vi "uc480_SimpleLive_MultiCamera.vi"() -> ()   [LabVIEW 2011]
uses:
  C:/Program Files/Thorlabs/Scientific Imaging/DCx Camera Support/Develop/DotNet/uc480DotNet.dll
  Develop/DotNet/uc480DotNet.dll
panel:
  in  "Init Camera 2":bool
  in  "Exit Camera 2":bool
  out "Error Out 2":errorcluster caption="error"
  out "Bits/Pixel 2":i32=8
  out "Width":i32=8
  out "Height Height 2":i32=8
  out "Serial Number 2":string
  in  "Camera ID 2":i32
  out "Image second camera":picture
  out "Image first camera":picture
  in  "Camera ID 1":i32
  out "Serial Number 1":string
  out "Height Height":i32=8
  out "Width":i32=8
  out "Bits/Pixel":i32=8
  out "Error Out 1":errorcluster caption="error"
  in  "Exit Camera":bool
  in  "Init Camera":bool
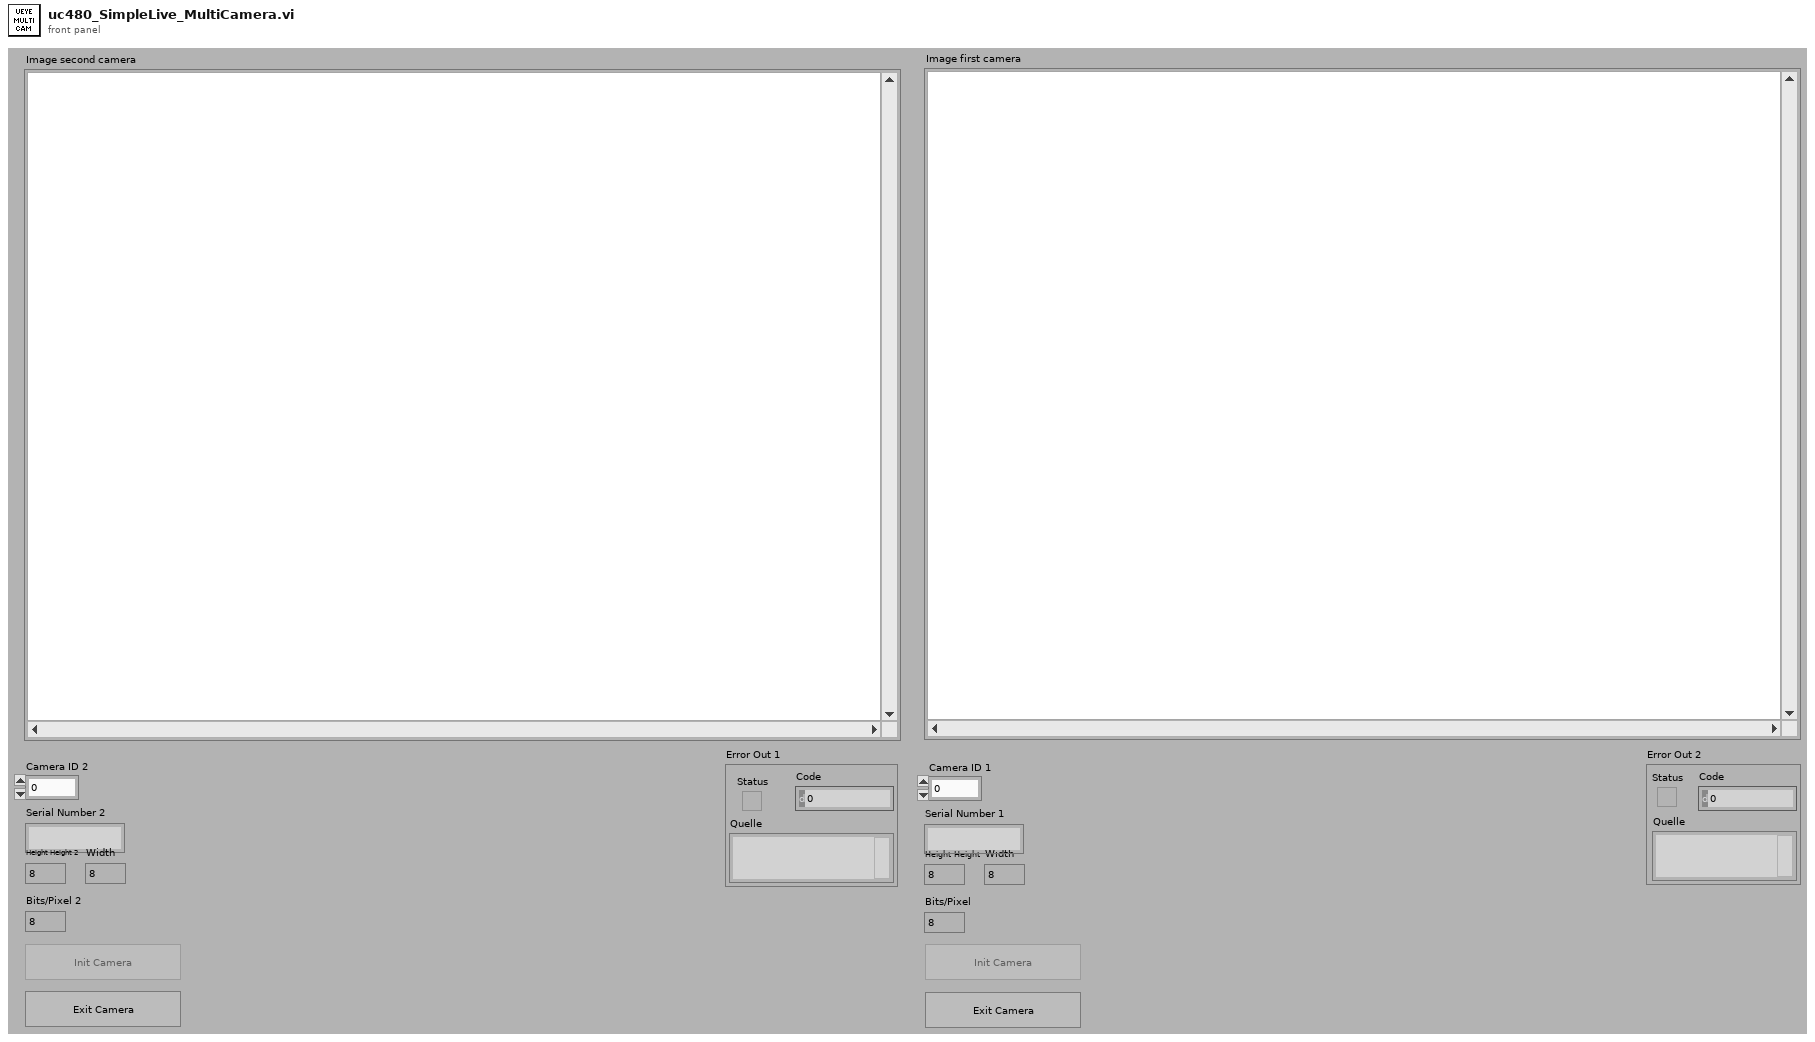
[diagram p1: front panel]
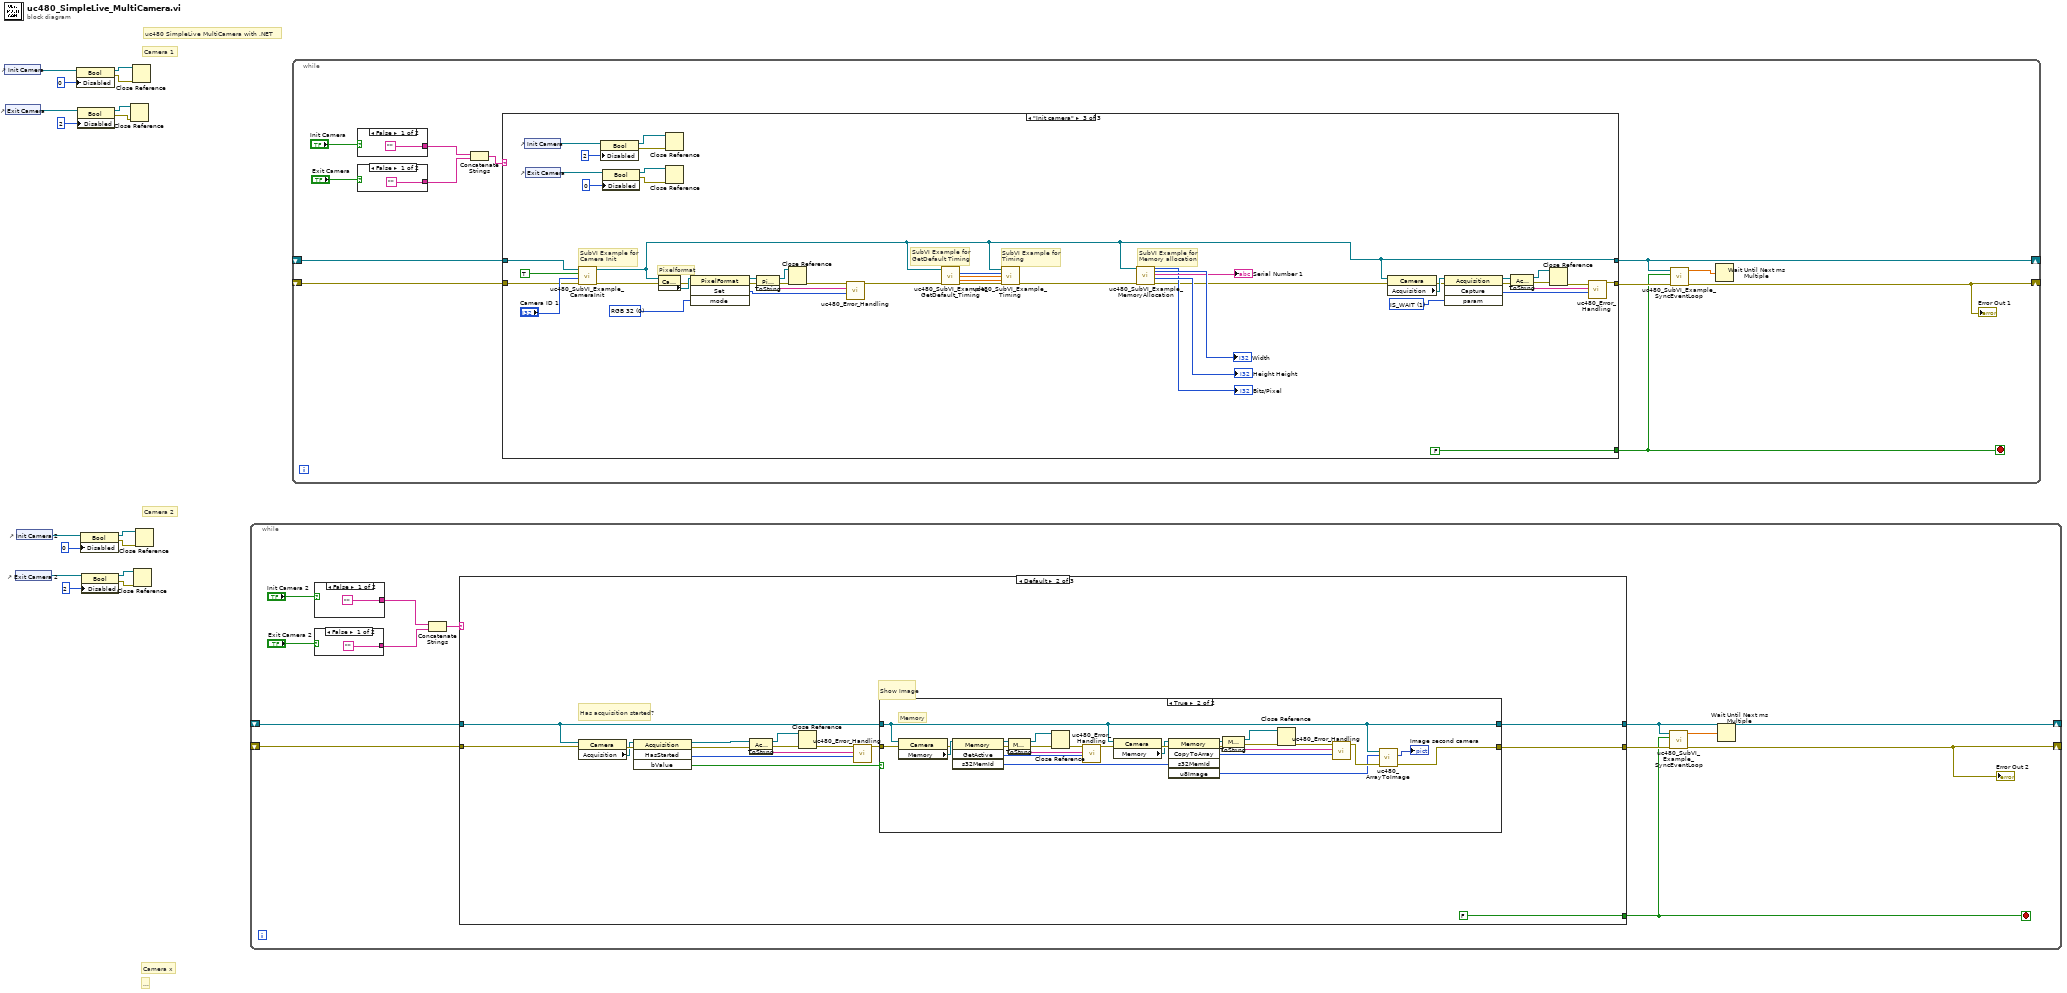
[diagram p0: block diagram]
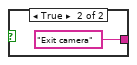
[diagram p2: hidden frame]
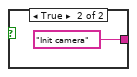
[diagram p3: hidden frame]
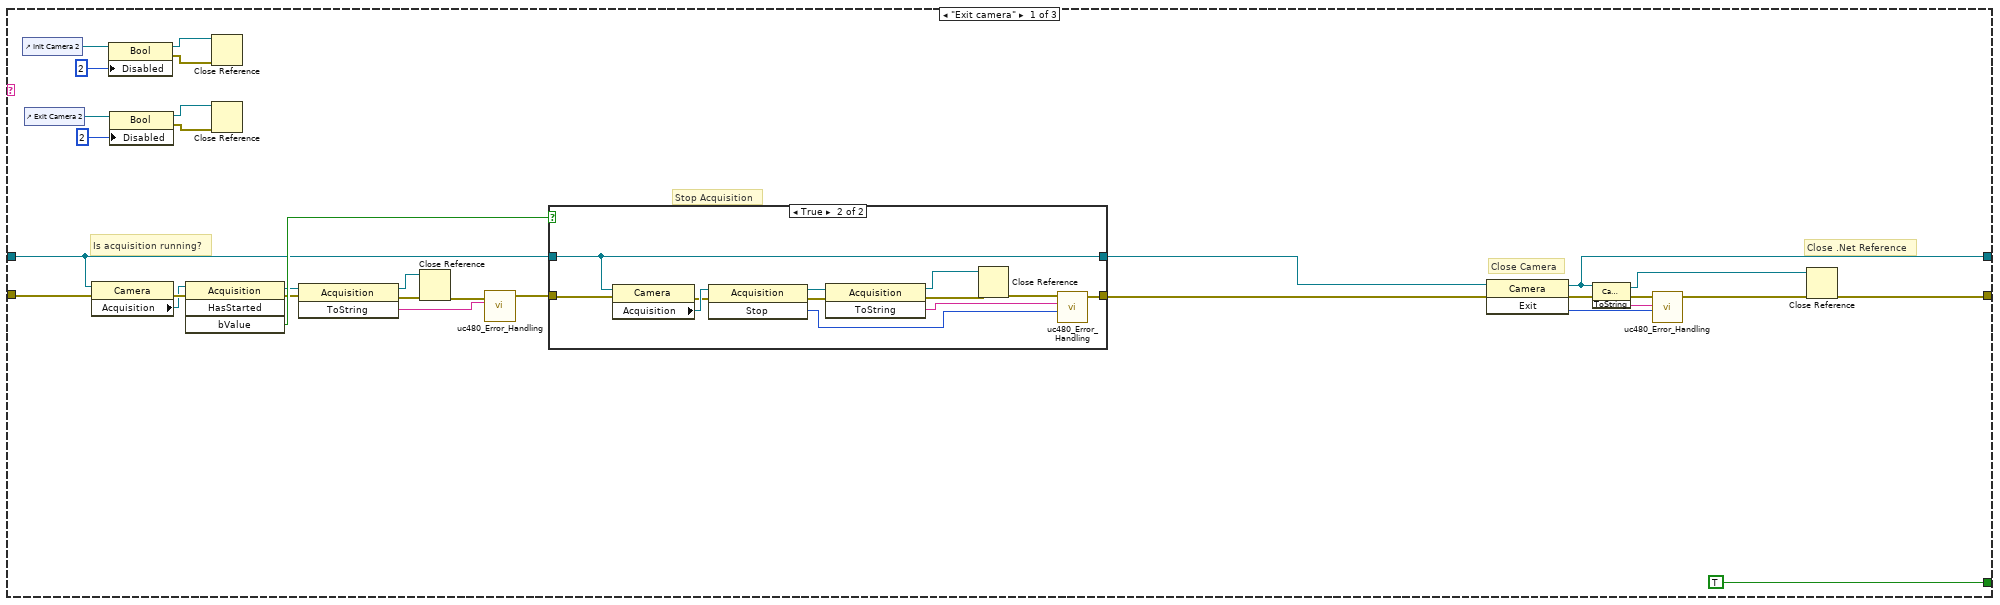
[diagram p4: hidden frame]
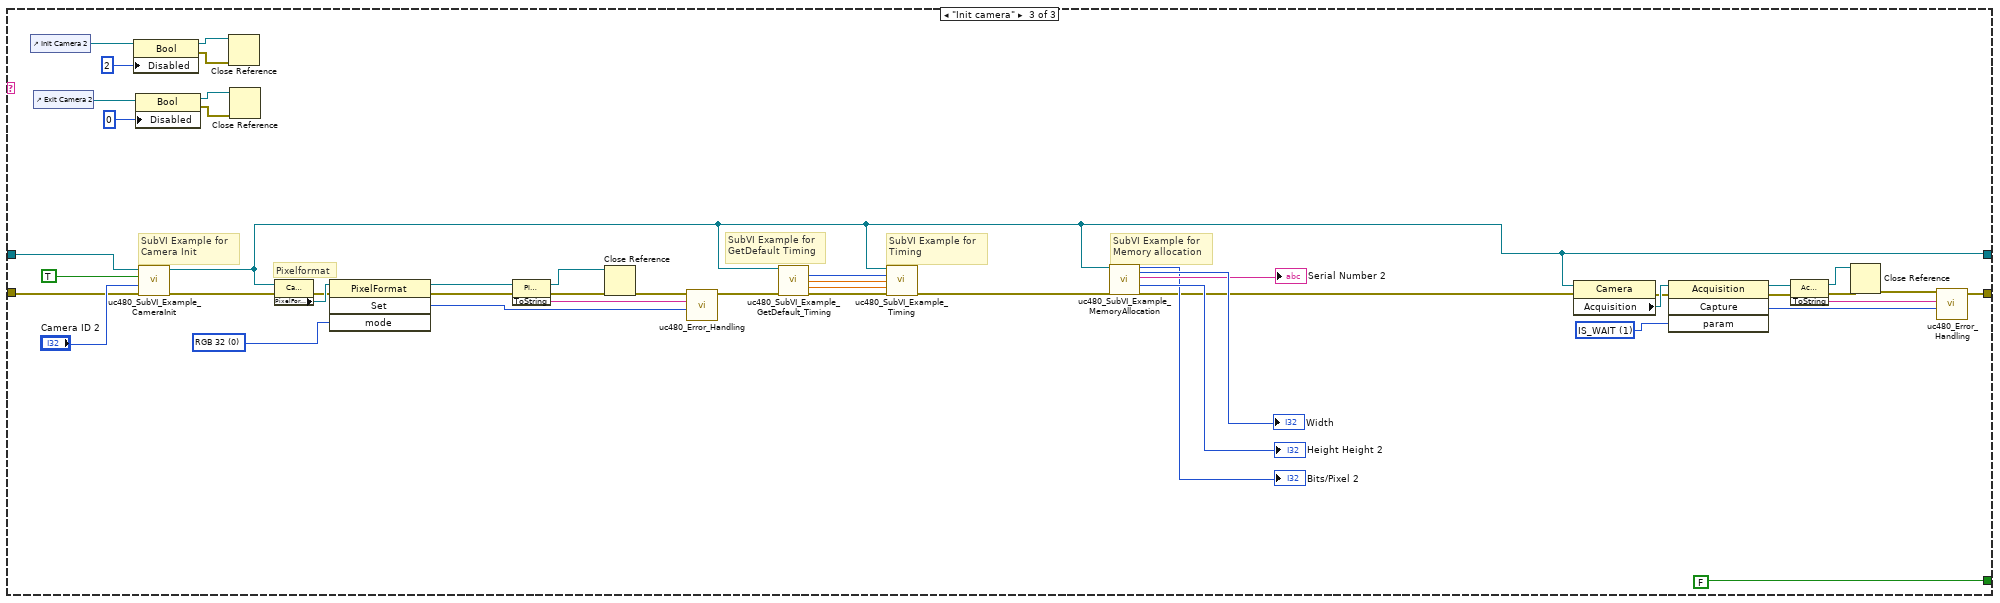
[diagram p7: hidden frame]
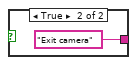
[diagram p8: hidden frame]
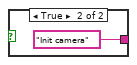
[diagram p9: hidden frame]
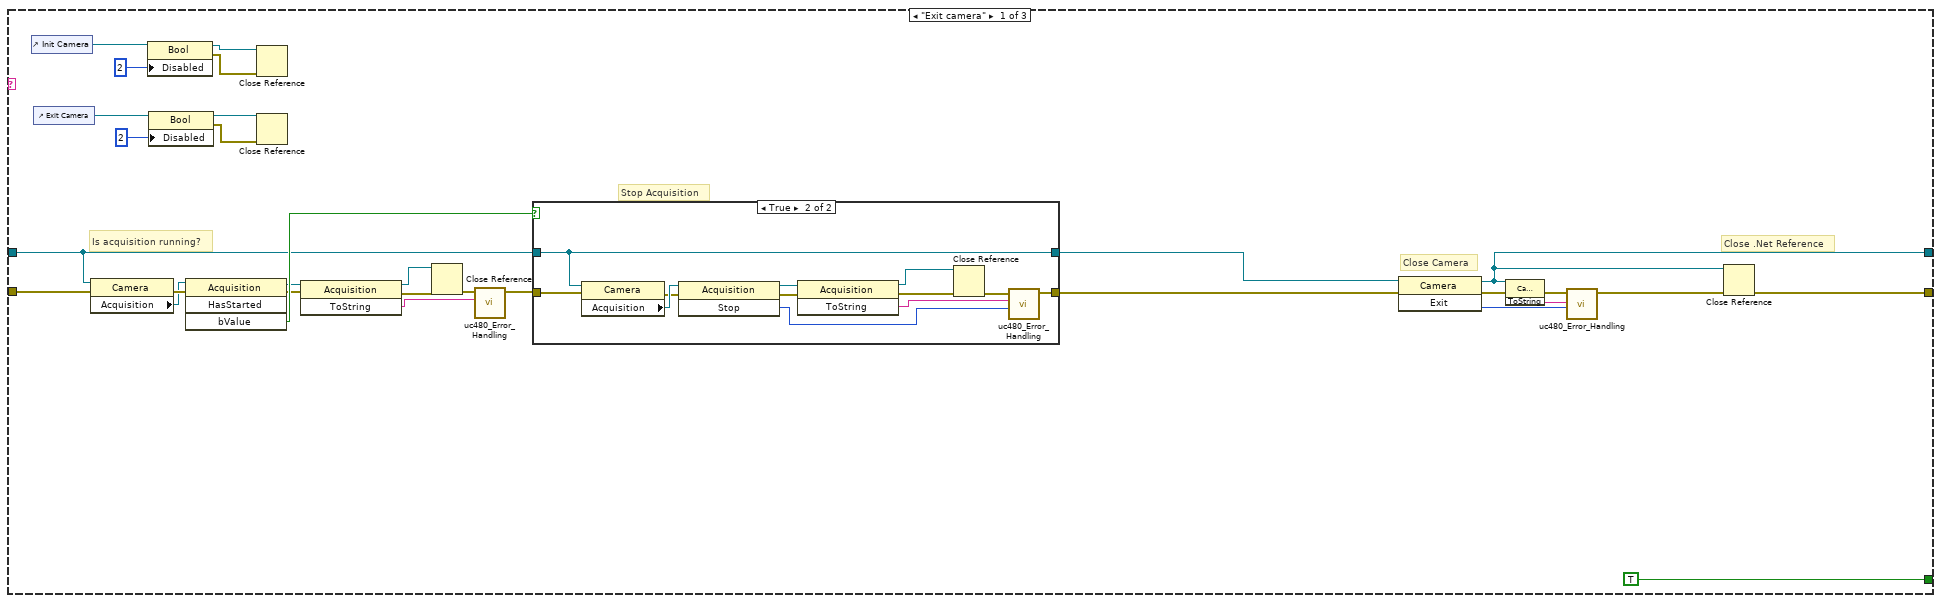
[diagram p10: hidden frame]
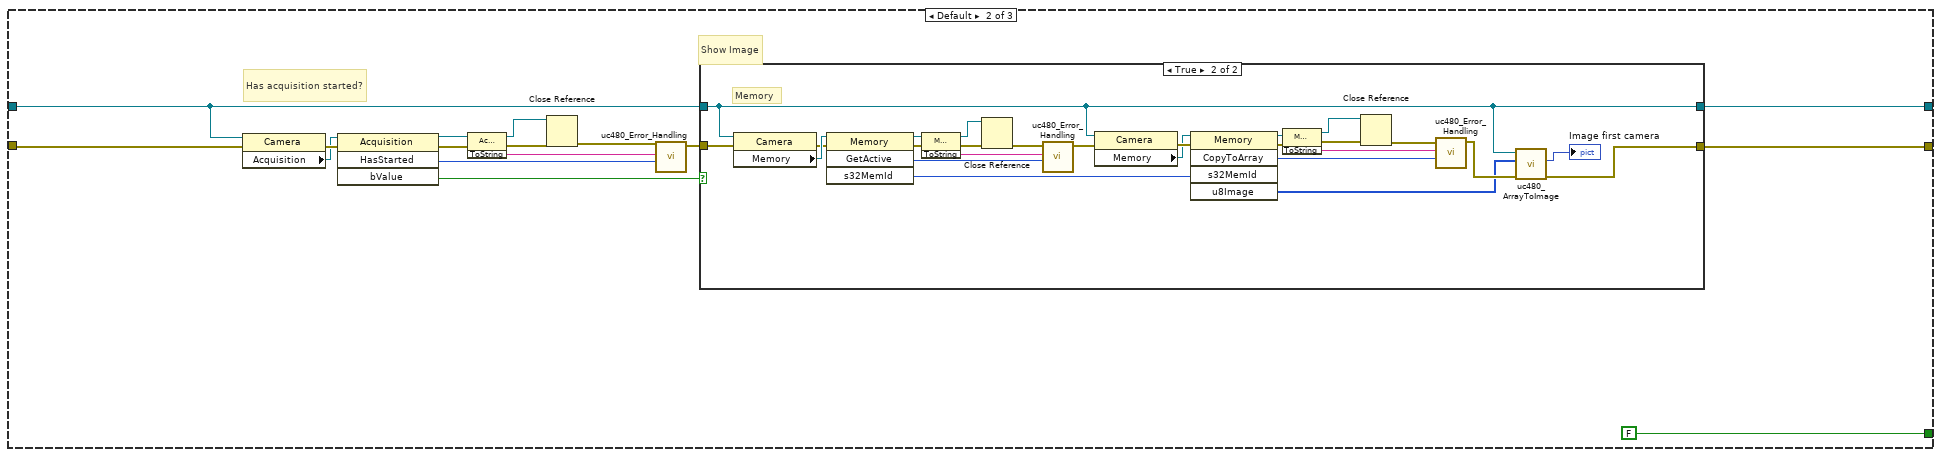
[diagram p12: hidden frame]
diagram:
  # "..."
  # "Camera x"
  # "Camera 2"
  # "Camera 1"
  # "uc480 SimpleLive MultiCamera with .NET"
  n1 = control-ref of="Init Camera"() -> (w14:refnum<vi>)
  n2 = control-ref of="Exit Camera"() -> (w13:refnum<vi>)
  n3 = control-ref of="Exit Camera 2"() -> (w9:refnum<vi>)
  n4 = control-ref of="Init Camera 2"() -> (w10:refnum<vi>)
  n5 = property class="Bool"(reference=w14, "Disabled"=u8 0 ("Deaktiviert")) -> (reference out=w8:refnum<vi>, error out=w7:errorcluster)  [unwired: 1 in]
  n6 = property class="Bool"(reference=w13, "Disabled"=u8 2 ("Deaktiviert")) -> (reference out=w6:refnum<vi>, error out=w5:errorcluster)  [unwired: 1 in]
  n7 = property class="Bool"(reference=w10, "Disabled"=u8 0 ("Deaktiviert")) -> (reference out=w4:refnum<vi>, error out=w3:errorcluster)  [unwired: 1 in]
  n8 = property class="Bool"(reference=w9, "Disabled"=u8 2 ("Deaktiviert")) -> (reference out=w2:refnum<vi>, error out=w1:errorcluster)  [unwired: 1 in]
  n9 = Close Reference ("Close Referenz")(reference=w6, error in (no error)=w5) -> ()  [unwired: 1 out]
  n10 = Close Reference ("Close Referenz")(reference=w8, error in (no error)=w7) -> ()  [unwired: 1 out]
  n11 = Close Reference ("Close Referenz")(reference=w2, error in (no error)=w1) -> ()  [unwired: 1 out]
  n12 = Close Reference ("Close Referenz")(reference=w4, error in (no error)=w3) -> ()  [unwired: 1 out]
  n13 = while {
    shift-right: [w19] -> _
    shift-left: _ -> [w23]
    shift-right: [w20] -> _
    shift-left: _ -> [w17]
    stop <- w18 stop-if-true
    n14 = case shown="False" "Exit Camera 2" {
      tunnel: ["" "Exit camera"] -> w24
      frame False {
      }
      frame True {
      }
    }
    n15 = case shown="False" "Init Camera 2" {
      tunnel: ["" "Init camera"] -> w27
      frame False {
      }
      frame True {
      }
    }
    n16 = Concatenate Strings(w27, w24) -> (w26:string)
    n17 = case shown="Default" w26 {
      tunnel: w17 -> [w47 w82 w160]
      tunnel: w23 -> [w48 w81 w159]
      tunnel: [w56 w84 w137] -> w20
      tunnel: [w57 w83 w138] -> w22
      tunnel: [TRUE FALSE FALSE] -> w18
      frame "Exit camera" {
        # "Close .Net Reference"
        # "Is acquisition running?"
        # "Stop Acquisition"
        # "Close Camera"
        n18 = control-ref of="Init Camera 2"() -> (w42:refnum<vi>)
        n19 = control-ref of="Exit Camera 2"() -> (w41:refnum<vi>)
        n20 = property class="Camera"(reference=w47, error in=w48) -> (error out=w55:errorcluster, "Acquisition"=w54:refnum<k24>)  [unwired: 1 out]
        n21 = property class="Bool"(reference=w42, "Disabled"=u8 2 ("Deaktiviert")) -> (reference out=w36:refnum<vi>, error out=w35:errorcluster)  [unwired: 1 in]
        n22 = property class="Bool"(reference=w41, "Disabled"=u8 2 ("Deaktiviert")) -> (reference out=w34:refnum<vi>, error out=w33:errorcluster)  [unwired: 1 in]
        n23 = invoke class="Acquisition" method="HasStarted"(reference=w54, error in=w55) -> (reference out=w49:refnum<k24>, error out=w51:errorcluster, "bValue"=w53:bool)  [unwired: 2 in, 1 out]
        n24 = Close Reference ("Close Referenz")(reference=w36, error in (no error)=w35) -> ()  [unwired: 1 out]
        n25 = Close Reference ("Close Referenz")(reference=w34, error in (no error)=w33) -> ()  [unwired: 1 out]
        n26 = invoke class="Acquisition" method="ToString"(reference=w49, error in=w51) -> (reference out=w37:refnum<k24>, error out=w39:errorcluster, "ToString"=w50:string)  [unwired: 1 in]
        n27 = Close Reference(reference=w37, error in (no error)=w39) -> (error out=w38:errorcluster)
        n28 = call "uc480_Error_Handling.vi"("Error String"=w50, "Error In"=w38) -> ("Error Out"=w52:errorcluster)  [unwired: 9 in]
        n29 = case shown="True" w53 {
          tunnel: [w65 w76] -> w45
          tunnel: w52 -> [w65 w77]
          tunnel: w47 -> [w64 w69]
          tunnel: [w64 w69] -> w46
          frame False {
          }
          frame True {
            n30 = property class="Camera"(reference=w69, error in=w77) -> (error out=w73:errorcluster, "Acquisition"=w74:refnum<k24>)  [unwired: 1 out]
            n31 = invoke class="Acquisition" method="Stop"(reference=w74, error in=w73) -> (reference out=w71:refnum<k24>, error out=w72:errorcluster, "Stop"=w70:i32)  [unwired: 1 in]
            n32 = invoke class="Acquisition" method="ToString"(reference=w71, error in=w72) -> (reference out=w66:refnum<k24>, error out=w68:errorcluster, "ToString"=w75:string)  [unwired: 1 in]
            n33 = Close Reference(reference=w66, error in (no error)=w68) -> (error out=w67:errorcluster)
            n34 = call "uc480_Error_Handling.vi"("Error Code"=w70, "Error String"=w75, "Error In"=w67) -> ("Error Out"=w76:errorcluster)  [unwired: 8 in]
          }
        }
        n35 = invoke class="Camera" method="Exit"(reference=w46, error in=w45) -> (reference out=w56:refnum<k24>, error out=w60:errorcluster, "Exit"=w59:i32)  [unwired: 1 in]
        n36 = invoke class="Camera" method="ToString"(reference=w56, error in=w60) -> (reference out=w40:refnum<k24>, error out=w61:errorcluster, "ToString"=w62:string)  [unwired: 1 in]
        n37 = call "uc480_Error_Handling.vi"("Error Code"=w59, "Error String"=w62, "Error In"=w61) -> ("Error Out"=w58:errorcluster)  [unwired: 8 in]
        n38 = Close Reference ("Close Referenz")(reference=w40, error in (no error)=w58) -> (error out=w57:errorcluster)
      }
      frame Default {
        # "Has acquisition started?"
        # "Show Image"
        n39 = property class="Camera"(reference=w82, error in=w81) -> (error out=w92:errorcluster, "Acquisition"=w91:refnum<k24>)  [unwired: 1 out]
        n40 = invoke class="Acquisition" method="HasStarted"(reference=w91, error in=w92) -> (reference out=w88:refnum<k24>, error out=w87:errorcluster, "HasStarted"=w86:i32, "bValue"=w90:bool)  [unwired: 2 in]
        n41 = invoke class="Acquisition" method="ToString"(reference=w88, error in=w87) -> (reference out=w78:refnum<k24>, error out=w80:errorcluster, "ToString"=w89:string)  [unwired: 1 in]
        n42 = Close Reference(reference=w78, error in (no error)=w80) -> (error out=w79:errorcluster)
        n43 = call "uc480_Error_Handling.vi"("Error Code"=w86, "Error String"=w89, "Error In"=w79) -> ("Error Out"=w85:errorcluster)  [unwired: 8 in]
        n44 = case shown="True" w90 {
          tunnel: [w95 w107] -> w83
          tunnel: w85 -> [w95 w106]
          tunnel: w82 -> [w94 w102]
          tunnel: [w94 w102] -> w84
          frame False {
          }
          frame True {
            # "Memory"
            n45 = property class="Camera"(reference=w102, error in=w106) -> (error out=w109:errorcluster, "Memory"=w110:refnum<k24>)  [unwired: 1 out]
            n46 = invoke class="Memory" method="GetActive"(reference=w110, error in=w109) -> (reference out=w115:refnum<k24>, error out=w114:errorcluster, "GetActive"=w116:i32, "s32MemId"=w108:i32)  [unwired: 2 in]
            n47 = invoke class="Memory" method="ToString"(reference=w115, error in=w114) -> (reference out=w99:refnum<k24>, error out=w101:errorcluster, "ToString"=w113:string)  [unwired: 1 in]
            n48 = Close Reference(reference=w99, error in (no error)=w101) -> (error out=w100:errorcluster)
            n49 = call "uc480_Error_Handling.vi"("Error Code"=w116, "Error String"=w113, "Error In"=w100) -> ("Error Out"=w117:errorcluster)  [unwired: 8 in]
            n50 = property class="Camera"(reference=w102, error in=w117) -> (error out=w112:errorcluster, "Memory"=w111:refnum<k24>)  [unwired: 1 out]
            n51 = invoke class="Memory" method="CopyToArray"(reference=w111, error in=w112, "s32MemId"=w108) -> (reference out=w119:refnum<k24>, error out=w120:errorcluster, "CopyToArray"=w121:i32, "u8Image"=w103:u8[])  [unwired: 2 in, 1 out]
            n52 = invoke class="Memory" method="ToString"(reference=w119, error in=w120) -> (reference out=w96:refnum<k24>, error out=w98:errorcluster, "ToString"=w118:string)  [unwired: 1 in]
            n53 = Close Reference(reference=w96, error in (no error)=w98) -> (error out=w97:errorcluster)
            n54 = call "uc480_Error_Handling.vi"("Error Code"=w121, "Error String"=w118, "Error In"=w97) -> ("Error Out"=w104:errorcluster)  [unwired: 8 in]
            n55 = call "uc480_ArrayToImage.vi"("Error In"=w104, "InArray"=w103, ".NET (Reference)"=w102) -> ("Error Out"=w107:errorcluster, "Image"=→"Image second camera":picture)  [unwired: 7 in]
          }
        }
      }
      frame "Init camera" {
        w139 = 1 items=["IS_DONT_WAIT", "IS_WAIT"] ("Wait")
        w168 = 0 items=["RGB 32"=0, "RGB 24"=1, "Y8 Monochrom"=6] ("Mode")
        # "SubVI Example for \nGetDefault Timing"
        # "SubVI Example for \nMemory allocation"
        # "SubVI Example for \nTiming"
        # "SubVI Example for \nCamera Init"
        # "Pixelformat"
        n56 = control-ref of="Init Camera 2"() -> (w134:refnum<vi>)
        n57 = control-ref of="Exit Camera 2"() -> (w132:refnum<vi>)
        n58 = property class="Bool"(reference=w134, "Disabled"=u8 2 ("Deaktiviert")) -> (reference out=w125:refnum<vi>, error out=w124:errorcluster)  [unwired: 1 in]
        n59 = property class="Bool"(reference=w132, "Disabled"=u8 0 ("Deaktiviert")) -> (reference out=w123:refnum<vi>, error out=w122:errorcluster)  [unwired: 1 in]
        n60 = call "uc480_SubVI_Example_CameraInit.vi"("Error In"=w159, "Camera ID"="Camera ID 2", "Init Camera Flag"=TRUE, ".NET (Reference)"=w160) -> ("Error Out"=w165:errorcluster, ".NET (Reference)"=w137:refnum<k24>)  [unwired: 6 in]
        n61 = Close Reference ("Close Referenz")(reference=w125, error in (no error)=w124) -> ()  [unwired: 1 out]
        n62 = Close Reference ("Close Referenz")(reference=w123, error in (no error)=w122) -> ()  [unwired: 1 out]
        n63 = property class="Camera"(reference=w137, error in=w165) -> (error out=w166:errorcluster, "PixelFormat"=w167:refnum<k24>)  [unwired: 1 out]
        n64 = invoke class="PixelFormat" method="Set"(reference=w167, error in=w166, "mode"=w168) -> (reference out=w163:refnum<k24>, error out=w156:errorcluster, "Set"=w162:i32)  [unwired: 1 in, 1 out]
        n65 = invoke class="PixelFormat" method="ToString"(reference=w163, error in=w156) -> (reference out=w129:refnum<k24>, error out=w131:errorcluster, "ToString"=w164:string)  [unwired: 1 in]
        n66 = Close Reference(reference=w129, error in (no error)=w131) -> (error out=w130:errorcluster)
        n67 = call "uc480_Error_Handling.vi"("Error Code"=w162, "Error String"=w164, "Error In"=w130) -> ("Error Out"=w150:errorcluster)  [unwired: 8 in]
        n68 = call "uc480_SubVI_Example_GetDefault_Timing.vi"(".NET (Reference)"=w137, "Error In"=w150) -> ("Pixelclock"=w147:i32, "Exposure time"=w148:dbl, "Framerate"=w149:dbl, "Error Out"=w146:errorcluster)  [unwired: 10 in]
        n69 = call "uc480_SubVI_Example_Timing.vi"(".NET (Reference)"=w137, "Pixelclock"=w147, "Exposure time"=w148, "Framerate"=w149, "Error In"=w146) -> ("Error Out"=w155:errorcluster)  [unwired: 7 in, 3 out]
        n70 = call "uc480_SubVI_Example_MemoryAllocation.vi"(".NET (Reference)"=w137, "Error In"=w155) -> ("Bits/Pixel 2"=→"Bits/Pixel 2":i32, "Width"=→"Width":i32, "Serial Number"=→"Serial Number 2":string, "Height"=→"Height Height 2":i32, "Error Out"=w136:errorcluster)  [unwired: 13 in]
        n71 = property class="Camera"(reference=w137, error in=w136) -> (error out=w144:errorcluster, "Acquisition"=w145:refnum<k24>)  [unwired: 1 out]
        n72 = invoke class="Acquisition" method="Capture"(reference=w145, error in=w144, "param"=w139) -> (reference out=w141:refnum<k24>, error out=w142:errorcluster, "Capture"=w140:i32)  [unwired: 1 in, 1 out]
        n73 = invoke class="Acquisition" method="ToString"(reference=w141, error in=w142) -> (reference out=w126:refnum<k24>, error out=w128:errorcluster, "ToString"=w143:string)  [unwired: 1 in]
        n74 = Close Reference(reference=w126, error in (no error)=w128) -> (error out=w127:errorcluster)
        n75 = call "uc480_Error_Handling.vi"("Error Code"=w140, "Error String"=w143, "Error In"=w127) -> ("Error Out"=w138:errorcluster)  [unwired: 8 in]
      }
    }
    n76 = call "uc480_SubVI_Example_SyncEventLoop.vi"("Error In"=w22, "use sync"=w18, ".NET (Reference)"=w20) -> ("Error Out"=w19:errorcluster, "Synchronize (ms)"=w21:dbl)  [unwired: 7 in]
    "Error Out 2" <- w19
    n77 = Wait Until Next ms Multiple(millisecond multiple=w21) -> ()  [unwired: 1 out]
  }
  n78 = while {
    shift-right: [w172] -> _
    shift-left: _ -> [w175]
    shift-right: [w173] -> _
    shift-left: _ -> [w169]
    stop <- w170 stop-if-true
    n79 = case shown="False" "Init Camera" {
      tunnel: ["" "Init camera"] -> w179
      frame False {
      }
      frame True {
      }
    }
    n80 = case shown="False" "Exit Camera" {
      tunnel: ["" "Exit camera"] -> w176
      frame False {
      }
      frame True {
      }
    }
    n81 = Concatenate Strings(w179, w176) -> (w178:string)
    n82 = case shown="\"Init camera\"" w178 {
      tunnel: w169 -> [w198 w233 w311]
      tunnel: w175 -> [w199 w232 w310]
      tunnel: [w207 w235 w289] -> w173
      tunnel: [w208 w234 w290] -> w174
      tunnel: [TRUE FALSE FALSE] -> w170
      frame "Exit camera" {
        # "Close .Net Reference"
        # "Is acquisition running?"
        # "Stop Acquisition"
        # "Close Camera"
        n83 = control-ref of="Init Camera"() -> (w193:refnum<vi>)
        n84 = control-ref of="Exit Camera"() -> (w192:refnum<vi>)
        n85 = property class="Camera"(reference=w198, error in=w199) -> (error out=w206:errorcluster, "Acquisition"=w205:refnum<k24>)  [unwired: 1 out]
        n86 = property class="Bool"(reference=w193, "Disabled"=u8 2 ("Deaktiviert")) -> (reference out=w188:refnum<vi>, error out=w187:errorcluster)  [unwired: 1 in]
        n87 = property class="Bool"(reference=w192, "Disabled"=u8 2 ("Deaktiviert")) -> (reference out=w186:refnum<vi>, error out=w185:errorcluster)  [unwired: 1 in]
        n88 = invoke class="Acquisition" method="HasStarted"(reference=w205, error in=w206) -> (reference out=w200:refnum<k24>, error out=w202:errorcluster, "bValue"=w204:bool)  [unwired: 2 in, 1 out]
        n89 = Close Reference ("Close Referenz")(reference=w188, error in (no error)=w187) -> ()  [unwired: 1 out]
        n90 = Close Reference ("Close Referenz")(reference=w186, error in (no error)=w185) -> ()  [unwired: 1 out]
        n91 = invoke class="Acquisition" method="ToString"(reference=w200, error in=w202) -> (reference out=w189:refnum<k24>, error out=w191:errorcluster, "ToString"=w201:string)  [unwired: 1 in]
        n92 = Close Reference(reference=w189, error in (no error)=w191) -> (error out=w190:errorcluster)
        n93 = call "uc480_Error_Handling.vi"("Error String"=w201, "Error In"=w190) -> ("Error Out"=w203:errorcluster)  [unwired: 9 in]
        n94 = case shown="True" w204 {
          tunnel: [w216 w227] -> w196
          tunnel: w203 -> [w216 w228]
          tunnel: w198 -> [w215 w220]
          tunnel: [w215 w220] -> w197
          frame False {
          }
          frame True {
            n95 = property class="Camera"(reference=w220, error in=w228) -> (error out=w224:errorcluster, "Acquisition"=w225:refnum<k24>)  [unwired: 1 out]
            n96 = invoke class="Acquisition" method="Stop"(reference=w225, error in=w224) -> (reference out=w222:refnum<k24>, error out=w223:errorcluster, "Stop"=w221:i32)  [unwired: 1 in]
            n97 = invoke class="Acquisition" method="ToString"(reference=w222, error in=w223) -> (reference out=w217:refnum<k24>, error out=w219:errorcluster, "ToString"=w226:string)  [unwired: 1 in]
            n98 = Close Reference(reference=w217, error in (no error)=w219) -> (error out=w218:errorcluster)
            n99 = call "uc480_Error_Handling.vi"("Error Code"=w221, "Error String"=w226, "Error In"=w218) -> ("Error Out"=w227:errorcluster)  [unwired: 8 in]
          }
        }
        n100 = invoke class="Camera" method="Exit"(reference=w197, error in=w196) -> (reference out=w207:refnum<k24>, error out=w211:errorcluster, "Exit"=w210:i32)  [unwired: 1 in]
        n101 = invoke class="Camera" method="ToString"(reference=w207, error in=w211) -> (error out=w212:errorcluster, "ToString"=w213:string)  [unwired: 1 in, 1 out]
        n102 = call "uc480_Error_Handling.vi"("Error Code"=w210, "Error String"=w213, "Error In"=w212) -> ("Error Out"=w209:errorcluster)  [unwired: 8 in]
        n103 = Close Reference ("Close Referenz")(reference=w207, error in (no error)=w209) -> (error out=w208:errorcluster)
      }
      frame Default {
        # "Has acquisition started?"
        # "Show Image"
        n104 = property class="Camera"(reference=w233, error in=w232) -> (error out=w243:errorcluster, "Acquisition"=w242:refnum<k24>)  [unwired: 1 out]
        n105 = invoke class="Acquisition" method="HasStarted"(reference=w242, error in=w243) -> (reference out=w239:refnum<k24>, error out=w238:errorcluster, "HasStarted"=w237:i32, "bValue"=w241:bool)  [unwired: 2 in]
        n106 = invoke class="Acquisition" method="ToString"(reference=w239, error in=w238) -> (reference out=w229:refnum<k24>, error out=w231:errorcluster, "ToString"=w240:string)  [unwired: 1 in]
        n107 = Close Reference(reference=w229, error in (no error)=w231) -> (error out=w230:errorcluster)
        n108 = call "uc480_Error_Handling.vi"("Error Code"=w237, "Error String"=w240, "Error In"=w230) -> ("Error Out"=w236:errorcluster)  [unwired: 8 in]
        n109 = case shown="True" w241 {
          tunnel: [w246 w258] -> w234
          tunnel: w236 -> [w246 w257]
          tunnel: w233 -> [w245 w255]
          tunnel: [w245 w255] -> w235
          frame False {
          }
          frame True {
            # "Memory"
            n110 = property class="Camera"(reference=w255, error in=w257) -> (error out=w260:errorcluster, "Memory"=w261:refnum<k24>)  [unwired: 1 out]
            n111 = invoke class="Memory" method="GetActive"(reference=w261, error in=w260) -> (reference out=w266:refnum<k24>, error out=w265:errorcluster, "GetActive"=w267:i32, "s32MemId"=w259:i32)  [unwired: 2 in]
            n112 = invoke class="Memory" method="ToString"(reference=w266, error in=w265) -> (reference out=w250:refnum<k24>, error out=w252:errorcluster, "ToString"=w264:string)  [unwired: 1 in]
            n113 = Close Reference(reference=w250, error in (no error)=w252) -> (error out=w251:errorcluster)
            n114 = call "uc480_Error_Handling.vi"("Error Code"=w267, "Error String"=w264, "Error In"=w251) -> ("Error Out"=w268:errorcluster)  [unwired: 8 in]
            n115 = property class="Camera"(reference=w255, error in=w268) -> (error out=w263:errorcluster, "Memory"=w262:refnum<k24>)  [unwired: 1 out]
            n116 = invoke class="Memory" method="CopyToArray"(reference=w262, error in=w263, "s32MemId"=w259) -> (reference out=w270:refnum<k24>, error out=w271:errorcluster, "CopyToArray"=w272:i32, "u8Image"=w254:u8[])  [unwired: 2 in, 1 out]
            n117 = invoke class="Memory" method="ToString"(reference=w270, error in=w271) -> (reference out=w247:refnum<k24>, error out=w249:errorcluster, "ToString"=w269:string)  [unwired: 1 in]
            n118 = Close Reference(reference=w247, error in (no error)=w249) -> (error out=w248:errorcluster)
            n119 = call "uc480_Error_Handling.vi"("Error Code"=w272, "Error String"=w269, "Error In"=w248) -> ("Error Out"=w256:errorcluster)  [unwired: 8 in]
            n120 = call "uc480_ArrayToImage.vi"("Error In"=w256, "InArray"=w254, ".NET (Reference)"=w255) -> ("Error Out"=w258:errorcluster, "Image"=→"Image first camera":picture)  [unwired: 7 in]
          }
        }
      }
      frame "Init camera" {
        w291 = 1 items=["IS_DONT_WAIT", "IS_WAIT"] ("Wait")
        w319 = 0 items=["RGB 32"=0, "RGB 24"=1, "Y8 Monochrom"=6] ("Mode")
        # "SubVI Example for \nGetDefault Timing"
        # "SubVI Example for \nMemory allocation"
        # "SubVI Example for \nTiming"
        # "SubVI Example for \nCamera Init"
        # "Pixelformat"
        n121 = control-ref of="Init Camera"() -> (w285:refnum<vi>)
        n122 = control-ref of="Exit Camera"() -> (w283:refnum<vi>)
        n123 = call "uc480_SubVI_Example_CameraInit.vi"("Error In"=w310, "Camera ID"="Camera ID 1", "Init Camera Flag"=TRUE, ".NET (Reference)"=w311) -> ("Error Out"=w316:errorcluster, ".NET (Reference)"=w289:refnum<k24>)  [unwired: 6 in]
        n124 = property class="Bool"(reference=w285, "Disabled"=u8 2 ("Deaktiviert")) -> (reference out=w276:refnum<vi>, error out=w275:errorcluster)  [unwired: 1 in]
        n125 = property class="Bool"(reference=w283, "Disabled"=u8 0 ("Deaktiviert")) -> (reference out=w274:refnum<vi>, error out=w273:errorcluster)  [unwired: 1 in]
        n126 = property class="Camera"(reference=w289, error in=w316) -> (error out=w317:errorcluster, "PixelFormat"=w318:refnum<k24>)  [unwired: 1 out]
        n127 = Close Reference ("Close Referenz")(reference=w276, error in (no error)=w275) -> ()  [unwired: 1 out]
        n128 = Close Reference ("Close Referenz")(reference=w274, error in (no error)=w273) -> ()  [unwired: 1 out]
        n129 = invoke class="PixelFormat" method="Set"(reference=w318, error in=w317, "mode"=w319) -> (reference out=w314:refnum<k24>, error out=w307:errorcluster, "Set"=w313:i32)  [unwired: 1 in, 1 out]
        n130 = invoke class="PixelFormat" method="ToString"(reference=w314, error in=w307) -> (reference out=w281:refnum<k24>, error out=w282:errorcluster, "ToString"=w315:string)  [unwired: 1 in]
        n131 = Close Reference(reference=w281, error in (no error)=w282) -> (error out=w280:errorcluster)
        n132 = call "uc480_Error_Handling.vi"("Error Code"=w313, "Error String"=w315, "Error In"=w280) -> ("Error Out"=w301:errorcluster)  [unwired: 8 in]
        n133 = call "uc480_SubVI_Example_GetDefault_Timing.vi"(".NET (Reference)"=w289, "Error In"=w301) -> ("Pixelclock"=w298:i32, "Exposure time"=w299:dbl, "Framerate"=w300:dbl, "Error Out"=w287:errorcluster)  [unwired: 10 in]
        n134 = call "uc480_SubVI_Example_Timing.vi"(".NET (Reference)"=w289, "Pixelclock"=w298, "Exposure time"=w299, "Framerate"=w300, "Error In"=w287) -> ("Error Out"=w306:errorcluster)  [unwired: 7 in, 3 out]
        n135 = call "uc480_SubVI_Example_MemoryAllocation.vi"(".NET (Reference)"=w289, "Error In"=w306) -> ("Bits/Pixel 2"=→"Bits/Pixel":i32, "Width"=→"Width":i32, "Serial Number"=→"Serial Number 1":string, "Height"=→"Height Height":i32, "Error Out"=w288:errorcluster)  [unwired: 13 in]
        n136 = property class="Camera"(reference=w289, error in=w288) -> (error out=w296:errorcluster, "Acquisition"=w297:refnum<k24>)  [unwired: 1 out]
        n137 = invoke class="Acquisition" method="Capture"(reference=w297, error in=w296, "param"=w291) -> (reference out=w293:refnum<k24>, error out=w294:errorcluster, "Capture"=w292:i32)  [unwired: 1 in, 1 out]
        n138 = invoke class="Acquisition" method="ToString"(reference=w293, error in=w294) -> (reference out=w277:refnum<k24>, error out=w279:errorcluster, "ToString"=w295:string)  [unwired: 1 in]
        n139 = Close Reference(reference=w277, error in (no error)=w279) -> (error out=w278:errorcluster)
        n140 = call "uc480_Error_Handling.vi"("Error Code"=w292, "Error String"=w295, "Error In"=w278) -> ("Error Out"=w290:errorcluster)  [unwired: 8 in]
      }
    }
    n141 = call "uc480_SubVI_Example_SyncEventLoop.vi"("Error In"=w174, "use sync"=w170, ".NET (Reference)"=w173) -> ("Error Out"=w172:errorcluster, "Synchronize (ms)"=w171:dbl)  [unwired: 7 in]
    "Error Out 1" <- w172
    n142 = Wait Until Next ms Multiple(millisecond multiple=w171) -> ()  [unwired: 1 out]
  }
